vi "WRITE EOL TESTFLAG FGV.vi"(7 "Enum":T1=enum."WRITE", 8 "error in (no error)":errorcluster, 10 "data":dbl[](array[numeric]) format="%.2f", 11 "signal list":refnum<k21>[](array[refnum])) -> (0 "error out":errorcluster)   [LabVIEW 2018]
uses:
  FGV States.ctl
  <vilib>/xnet/xnet.llb/XNET Write (Signal Single-point).vi
  <vilib>/xnet/xnet.llb/XNET Create Session (Signal Output Single-point).vi
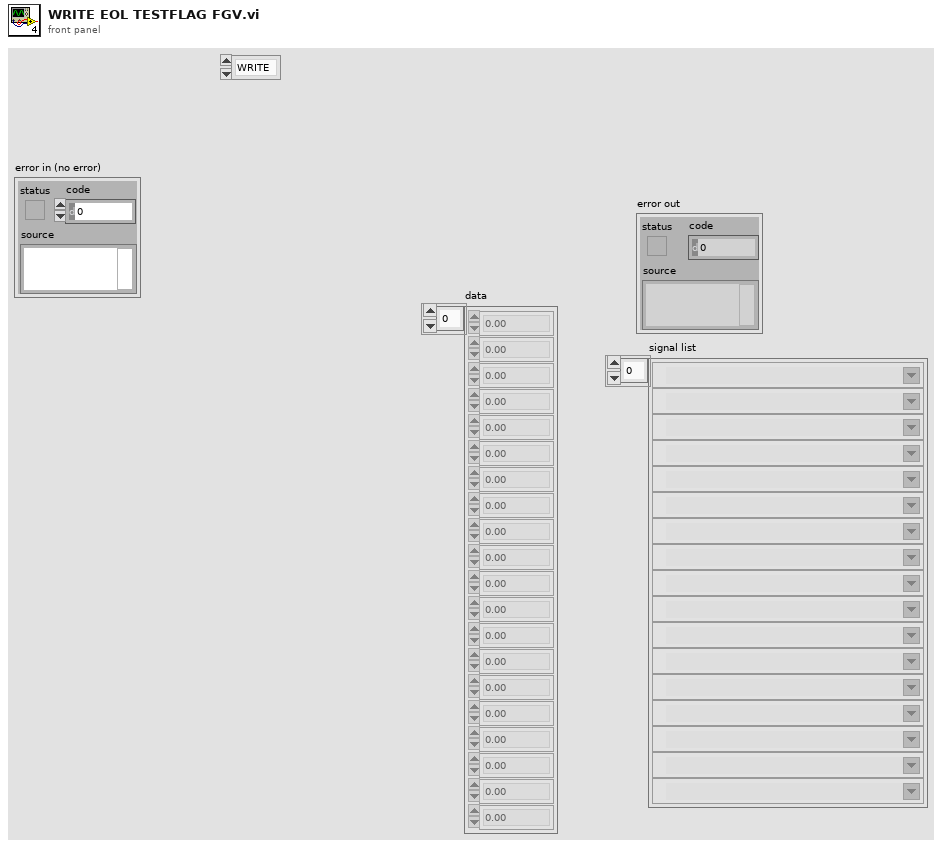
[diagram p1: front panel]
types:
  T1 = typedef "FGV States.ctl" = enum16{"OPEN", "READ", "CLOSE", "WRITE"}
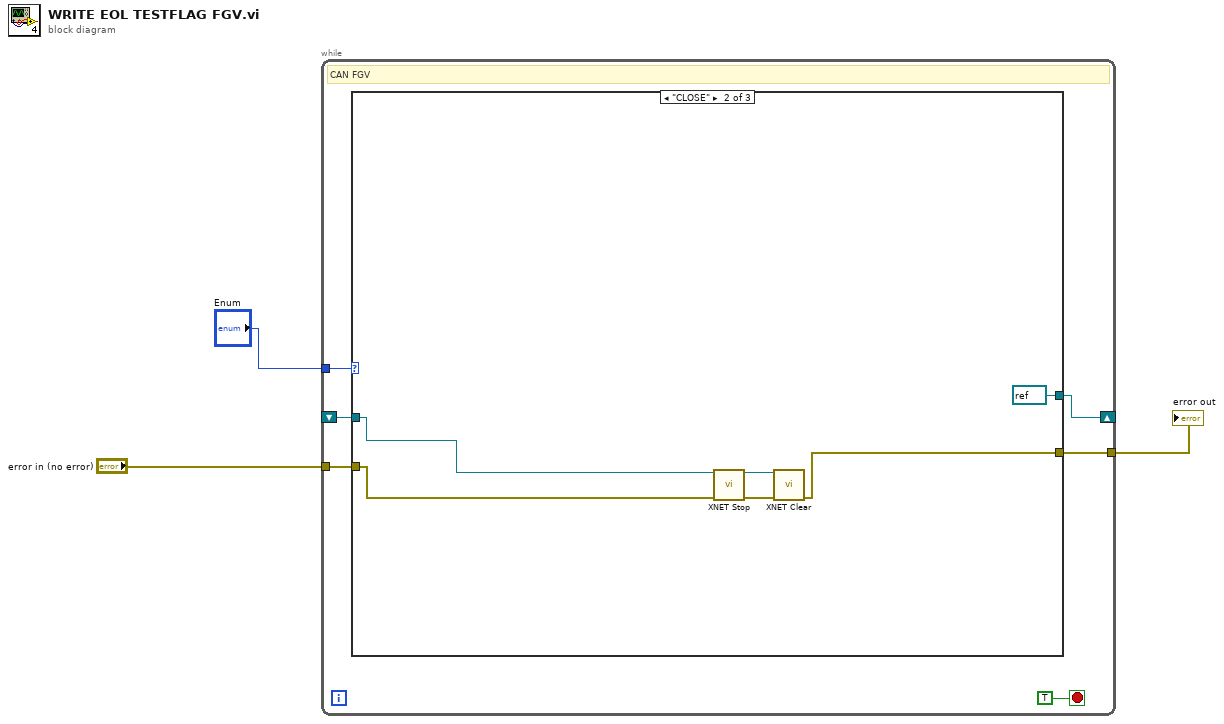
[diagram p0: block diagram]
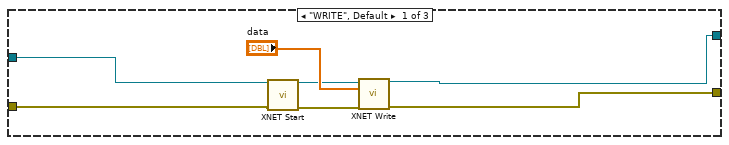
[diagram p2: hidden frame]
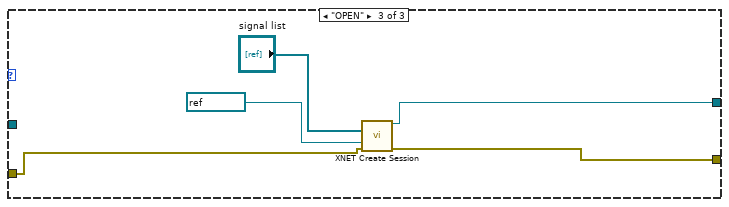
[diagram p3: hidden frame]
diagram:
  n1 = while {
    tunnel: "Enum" -> [w8]
    shift-right: [w7] -> _
    shift-left: _ -> [w6]
    tunnel: [w5] -> w1
    tunnel: "error in (no error)" -> [w4]
    stop <- TRUE stop-if-true
    # "CAN FGV"
    n2 = case shown="\"CLOSE\"" w8 {
      tunnel: [w15 refnum<k21> refnum ("session out") w23] -> w7
      tunnel: w6 -> [w11 w18 _]
      tunnel: [w16 w19 w24] -> w5
      tunnel: w4 -> [w13 w20 w25]
      frame "WRITE", Default {
        n3 = call <vilib>:"XNET Start.vi"("session in"=w11, "error in (no error)"=w13) -> ("session out"=w10:refnum<k21>, "error out"=w12:errorcluster)  [unwired: 12 in]
        n4 = call-poly <vilib>:"XNET Write.vi"("session in"=w10, "data"="data", "error in (no error)"=w12) -> ("session out"=w15:refnum<k21>, "error out"=w16:errorcluster)  [unwired: 11 in]
      }
      frame "CLOSE" {
        n5 = call <vilib>:"XNET Stop.vi"("session in"=w18, "error in (no error)"=w20) -> ("session out"=w21:refnum<k21>, "error out"=w22:errorcluster)  [unwired: 12 in]
        n6 = call <vilib>:"XNET Clear.vi"("session in"=w21, "error in (no error)"=w22) -> ("error out"=w19:errorcluster)  [unwired: 13 in]
      }
      frame "OPEN" {
        n7 = call-poly <vilib>:"XNET Create Session.vi"("signal list"="signal list", "interface"=refnum<k21> "CAN1" ("Select Interface"), "error in (no error)"=w25) -> ("session out"=w23:refnum<k21>, "error out"=w24:errorcluster)  [unwired: 11 out]
      }
    }
  }
  "error out" <- w1
